vi "KeyenceScan.vi"(8 "Error In":errorcluster, 9 "Timeout (ms)":i32, 10 "SN Length":i32, 11 "COM":string) -> (0 "Error Out":errorcluster, 2 "Read":string, 3 "NoScan":bool)   [LabVIEW 2016, in "MC2.lvlib"]
uses:
  MC2.lvlib
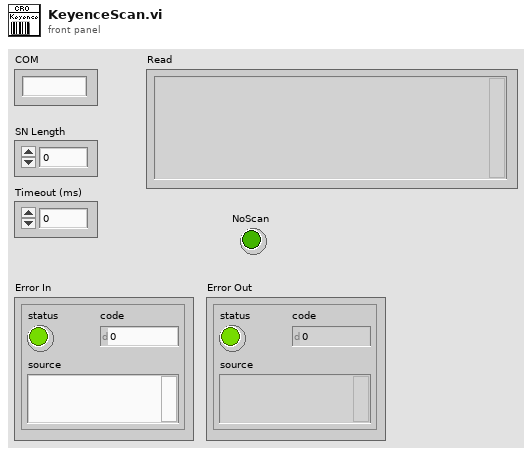
[diagram p1: front panel]
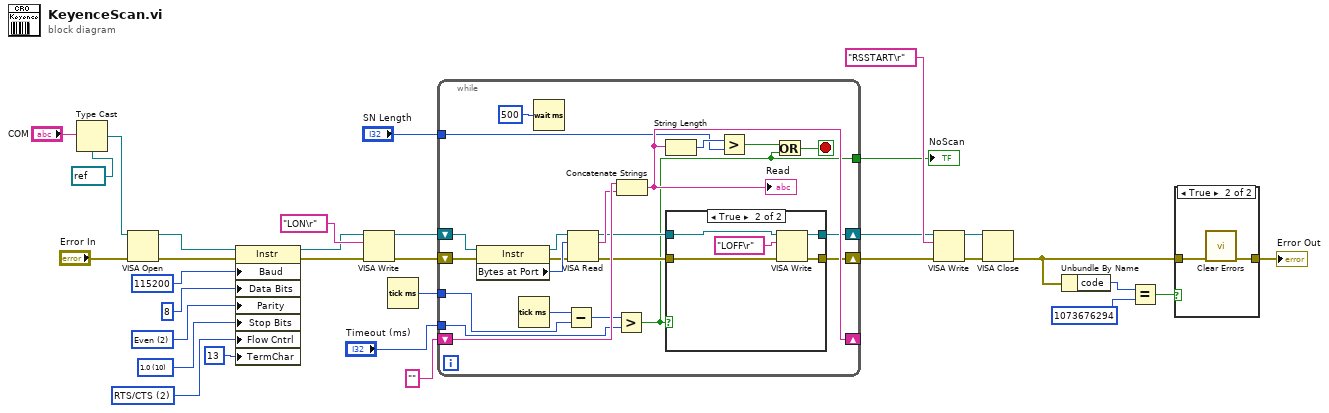
[diagram p0: block diagram]
diagram:
  w27 = u16 2 items=["None", "XON/XOFF", "RTS/CTS", "XON/XOFF & RTS/CTS", "DTR/DSR", "XON/XOFF & DTR/DSR"] ("Serial Settings:Flow Control")
  w29 = u16 10 items=["1.0"=10, "1.5"=15, "2.0"=20] ("Serial Settings:Stop Bits")
  w30 = u16 2 items=["None", "Odd", "Even", "Mark", "Space"] ("Serial Settings:Parity")
  n1 = Type Cast(type=refnum<visa-resource-name> refnum ("COM"), x="COM") -> (*(type *) &x=w6:refnum<visa-resource-name>)
  n2 = VISA Open(error in (no error)="Error In", VISA resource name=w6) -> (VISA resource name=w24:refnum<visa-resource-name>, error out=w22:errorcluster)  [unwired: 3 in]
  n3 = property class="Instr"(reference=w24, error in=w22, "Baud"=u32 115200 ("Serial Settings:Baud Rate"), "Data Bits"=u16 8 ("Serial Settings:Data Bits"), "Parity"=w30, "Stop Bits"=w29, "Flow Cntrl"=w27, "TermChar"=u8 13 ("Message Based Settings:Termination Character")) -> (reference out=w17:refnum<visa-resource-name>, error out=w16:errorcluster)
  n4 = VISA Write(VISA resource name=w17, write buffer="LON\r", error in (no error)=w16) -> (VISA resource name out=w19:refnum<visa-resource-name>, error out=w20:errorcluster)  [unwired: 1 out]
  n5 = Tick Count (ms)() -> (millisecond timer value=w11:u32)
  n6 = while {
    shift-right: [w34] -> w15
    shift-left: w19 -> [w50]
    shift-right: [w36] -> w14
    shift-left: w20 -> [w51]
    shift-right: [w46] -> _
    shift-left: "" -> [w49]
    tunnel: "SN Length" -> [w44]
    tunnel: w11 -> [w42]
    tunnel: "Timeout (ms)" -> [w40]
    tunnel: [w33] -> w9
    stop <- w38 stop-if-true
    n7 = property class="Instr"(reference=w50, error in=w51) -> (reference out=w54:refnum<visa-resource-name>, error out=w52:errorcluster, "Bytes at Port"=w53:u32)
    n8 = Tick Count (ms)() -> (millisecond timer value=w43:u32)
    n9 = Wait (ms)(milliseconds to wait=u32 500) -> ()  [unwired: 1 out]
    n10 = Subtract(x=w43, y=w42) -> (x-y=w41:u32)
    n11 = VISA Read(VISA resource name=w54, byte count=w53, error in (no error)=w52) -> (VISA resource name out=w35:refnum<visa-resource-name>, read buffer=w48:string, error out=w37:errorcluster)  [unwired: 1 out]
    n12 = Greater?(x=w41, y=w40) -> (0:w33:bool)
    n13 = Concatenate Strings(w49, w48) -> (w46:string)
    "Read" <- w46
    n14 = String Length(string=w46) -> (length=w45:i32)
    n15 = case shown="True" w33 {
      tunnel: w37 -> [w56 w61]
      tunnel: [w56 w57] -> w36
      tunnel: w35 -> [w55 w59]
      tunnel: [w55 w58] -> w34
      frame False {
      }
      frame True {
        n16 = VISA Write(VISA resource name=w59, write buffer="LOFF\r", error in (no error)=w61) -> (VISA resource name out=w58:refnum<visa-resource-name>, error out=w57:errorcluster)  [unwired: 1 out]
      }
    }
    n17 = Greater?(x=w45, y=w44) -> (0:w39:bool)
    n18 = Or(x=w39, y=w33) -> (x .or. y?=w38:bool)
  }
  "NoScan" <- w9
  n19 = VISA Write(VISA resource name=w15, write buffer="RSSTART\r", error in (no error)=w14) -> (VISA resource name out=w13:refnum<visa-resource-name>, error out=w12:errorcluster)  [unwired: 1 out]
  n20 = VISA Close(VISA resource name=w13, error in (no error)=w12) -> (error out=w2:errorcluster)
  n21 = Unbundle By Name(w2) -> ("code"=w5:i32)
  n22 = Equal?(x=w5, y=1073676294) -> (x = y?=w3:bool)
  n23 = case shown="True" w3 {
    tunnel: w2 -> [w62 w64]
    tunnel: [w62 w63] -> w1
    frame False {
    }
    frame True {
      n24 = call <vilib>:"Clear Errors.vi"("error in (no error)"=w64) -> ("error out"=w63:errorcluster)  [unwired: 5 in, 1 out]
    }
  }
  "Error Out" <- w1
